vi "RabiMeasurement.vi"() -> ()   [LabVIEW 2020]
uses:
  <vilib>/Swabian Instruments/Pulse Streamer/PulseStreamer/PulseStreamer/typedefs/typedef_TriggerStart.ctl
  <vilib>/Swabian Instruments/Pulse Streamer/PulseStreamer/PulsePattern/PulsePattern.lvclass
  C:/Program Files (x86)/National Instruments/LabVIEW 2020/vi.lib/Swabian Instruments/Pulse Streamer/PulseStreamer/Pattern/Pattern.lvclass
  <vilib>/Swabian Instruments/Pulse Streamer/PulseStreamer/typedefs/typedef_ChannelNumber.ctl
  <vilib>/Swabian Instruments/Pulse Streamer/PulseStreamer/AnalogPattern/AnalogPattern.lvclass
  <vilib>/Swabian Instruments/Pulse Streamer/PulseStreamer/Sequence/Sequence.lvclass/Sequence.ctl
  <vilib>/Analysis/baseanly.llb/Mean (DBL).vi
  <vilib>/FPGAPlugInAG/USB-7855R/niLvFpga_Open_USB-7855R.vi
  <vilib>/rvi/interface/common/dynamic/niFpgaDynamicAddResources.vi
  <vilib>/rvi/interface/common/niFpgaWaitOnOcc.vi
  <vilib>/Utility/error.llb/Error Cluster From Error Code.vi
  <vilib>/Swabian Instruments/Pulse Streamer/PulseStreamer/Pattern/Read total duration.vi
  <vilib>/Swabian Instruments/Pulse Streamer/PulseStreamer/PulseStreamer/stream/stream (Sequence).vi
  <vilib>/rvi/errors/niLvFpgaAdjustHostInterfaceError.vi
  <vilib>/FPGAPlugInAG/Dynamic/niLvFpga_Close_Dynamic.vi
  <vilib>/rvi/interface/nirviOpenFPGA/nirviOpenFPGA.xnode
  FPGA Bitfiles/pulsedcodespract_FPGATarget_FPGAReadout_kZLwuzG+bY8.lvbitx
  <vilib>/rvi/interface/nirviMethod/nirviMethod.xnode
  <vilib>/rvi/interface/nirviCloseFPGA/nirviCloseFPGA.xnode
  <vilib>/Swabian Instruments/Pulse Streamer/PulseStreamer/PulseStreamer/PulseStreamer.lvclass
  <vilib>/Swabian Instruments/Pulse Streamer/PulseStreamer/Sequence/Sequence.lvclass
  <vilib>/FPGAPlugInAG/Dynamic/niLvFpga_ConfigureFifo_Dynamic.vi
  <vilib>/rvi/errors/niLvFpgaMergeErrorWithErrorCode.vi
  <vilib>/Swabian Instruments/Pulse Streamer/PulseStreamer/PulseStreamer.lvlib
  <vilib>/FPGAPlugInAG/Dynamic/niLvFpga_ReadFifo_Dynamic.vi
  <vilib>/Analysis/NI_AALBase.lvlib
panel:
  in  "532 AOM Voltage":dbl min=-1.0 max=1.0
  in  "Pulser Start":T1
  out "Elements Remaining":dbl
  out "Cycle Num":i32
  in  "Delay(ns)":i32=760
  out "Seq Duration(ms)":dbl
  out "size(s)":dbl
  out "n_runs":i32
  out "Tau Set":i32
  out "Exp Number":i32
  in  "IP PulseBlaster":string="169.254.8.2"
  in  "Cycles":i32
  in  "Tau Step(ns)":i32=1
  in  "Tau Start(ns)":i32=5
  in  "Expt Repeat":u32=1000
  in  "Repeat":i32=10
  in  "Pulse Num":i32=100000
  in  "Wait Time(ns)":i32=600
  in  "Readout (ns)":i32=200
  in  "Initialization time (ns)":i32=1000
  out "ESR Plot Avg":cluster{"Tau":i32[], dbl[]}(graph)
  out "AvgCountsTrack":cluster{"Tau":i32[], dbl[]}(graph)
  out "Averaged_ESR":dbl[](array[numeric])
  out "AverageCounts This Run":cluster{"N_array":i32[], "CountAverage":dbl[]}(graph)
  out "Count_Track":dbl[](array[numeric])
  out "N_array":i32[](array[numeric])
  out "CountAverage":dbl[](array[numeric])
  out "ESR Plot Current Run":cluster{"Tau":i32[], "ESR Data":dbl[]}(graph)
  out "Counts":cluster{"Tau":i32[], "Count":u32[]}(graph)
  out "Tau":i32[](array[numeric])
  out "ESR Data":dbl[](array[numeric])
  out "Count":u32[](array[numeric])
  out "Digital plot":cluster{"CumTime":i64[], dbl[]}[](graph)
  out "RF Freq Set(GHz)":dbl format="%_8g"
  in  "RF Power (dBm)":dbl=1000000000.0 format="%_4g"
  in  "RF Freq(Hz)":dbl=1000000000.0 format="%_8g"
  in  "GPIB Reference":string="1:27"
  in  "?":bool
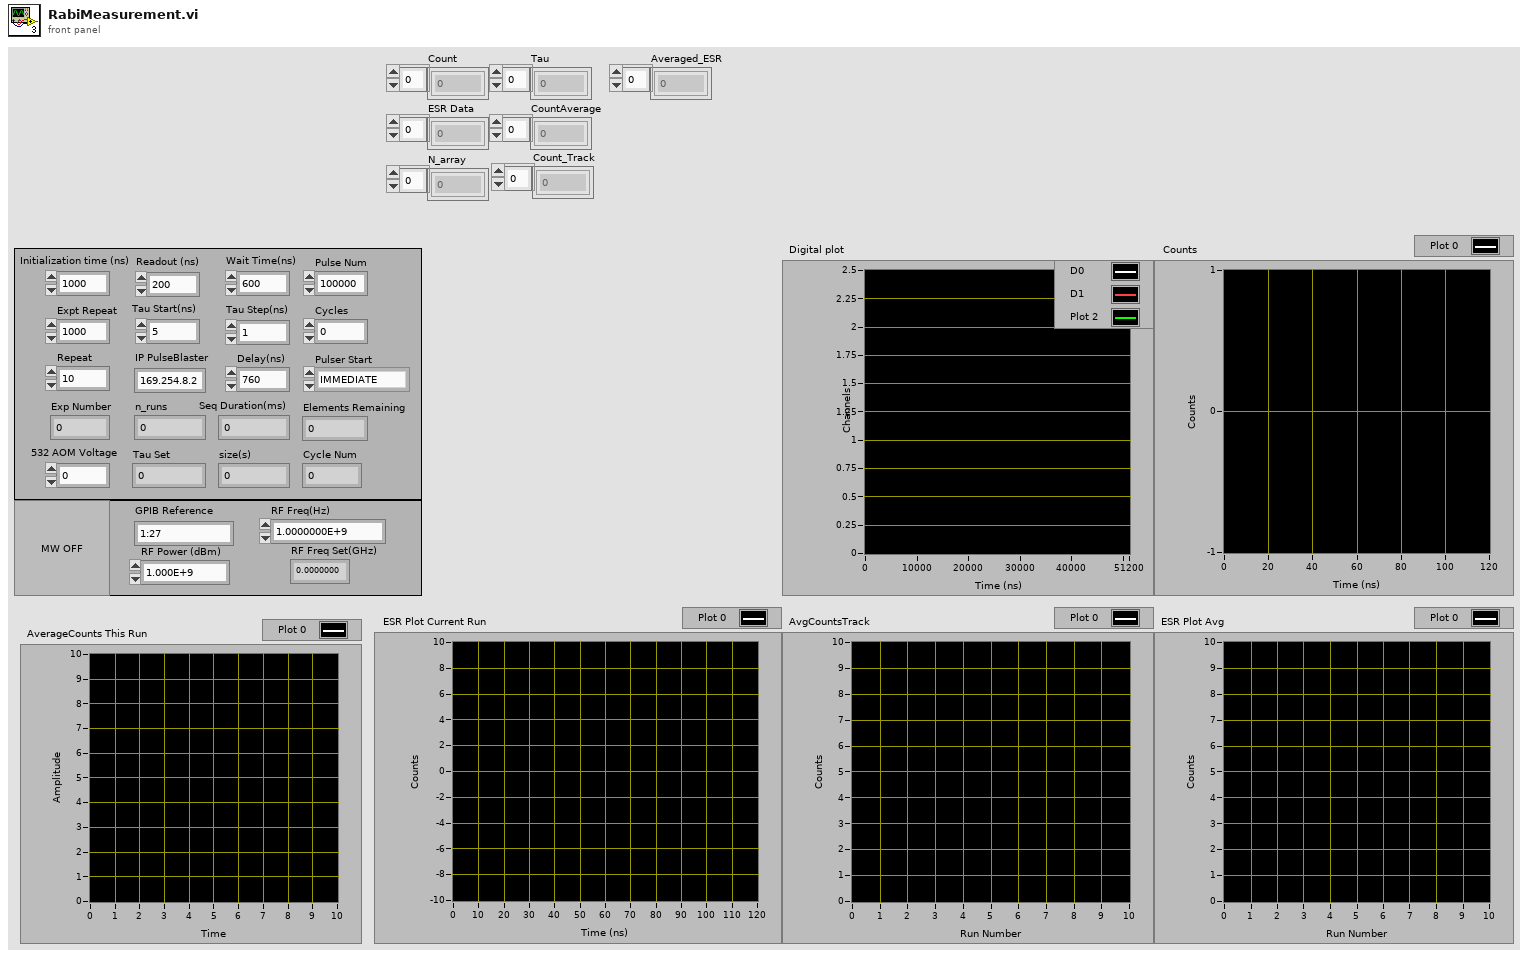
[diagram p1: front panel]
types:
  T1 = typedef "PulseStreamer.lvlib/PulseStreamer.lvclass/typedef_TriggerStart.ctl" = enum16{"IMMEDIATE", "SOFTWARE", "HW_RISING", "HW_FALLING", "HW_RISING_AND_FALLING"}
  T2 = typedef "PulseStreamer.lvlib/typedef_ChannelNumber.ctl" = i16
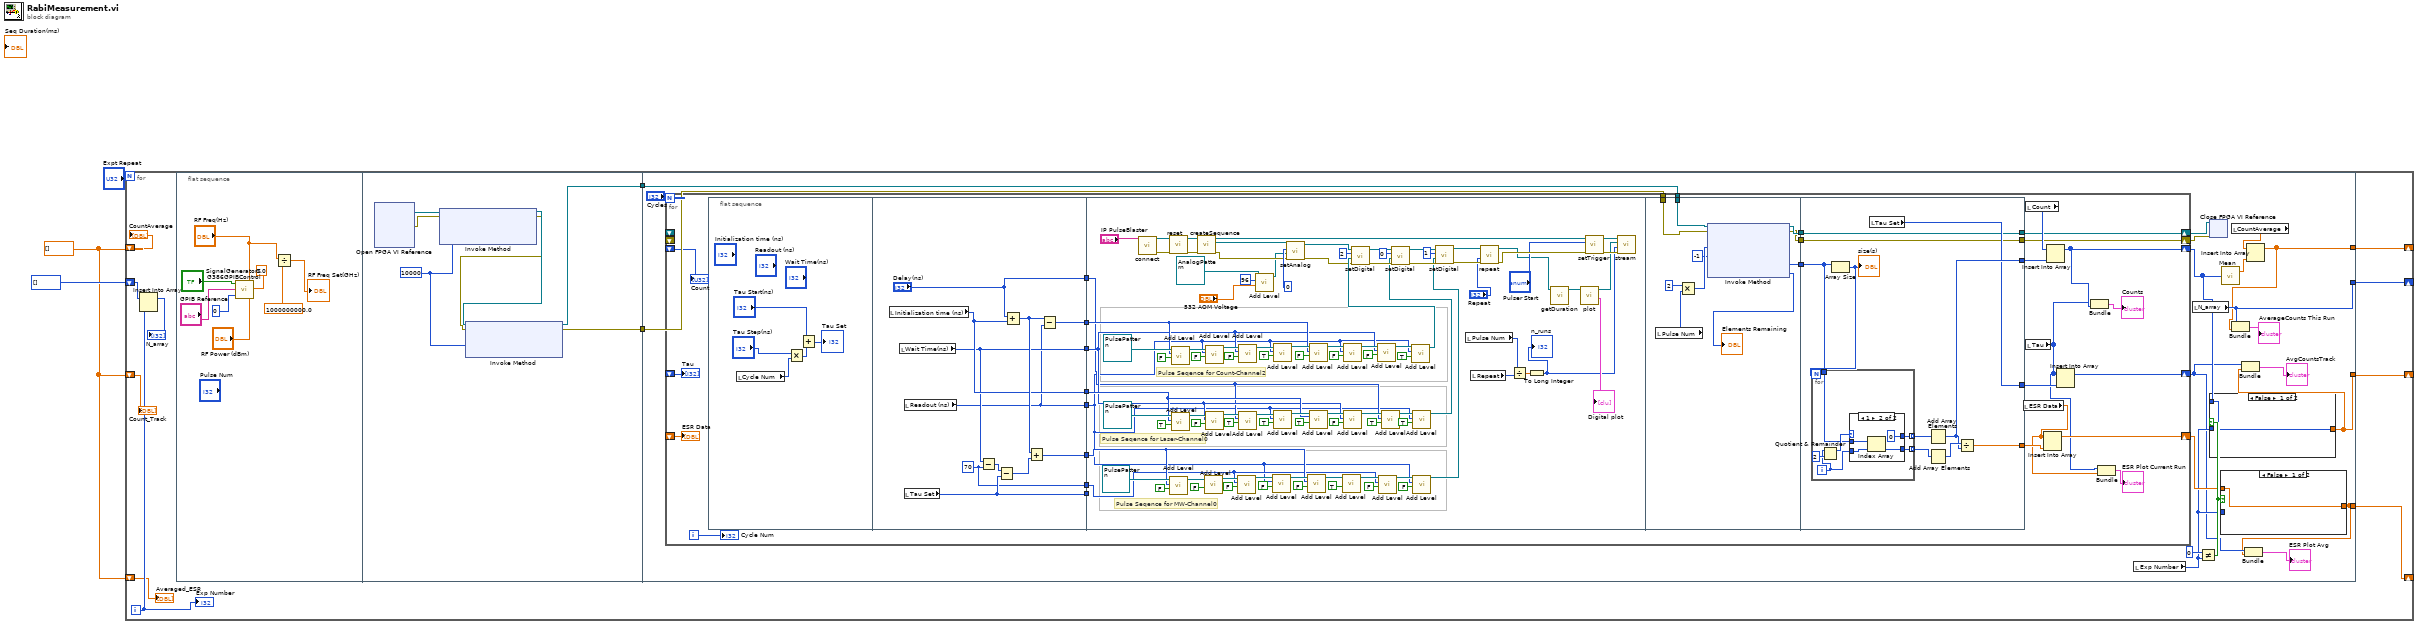
[diagram p0: block diagram]
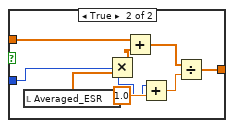
[diagram p2: hidden frame]
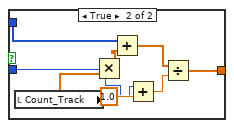
[diagram p3: hidden frame]
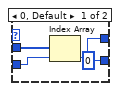
[diagram p4: hidden frame]
diagram:
  w1 = dbl[] []
  n1 = for {
    N: "Expt Repeat" -> [_]
    shift-right: [w13] -> _
    shift-left: w1 -> [w12]
    shift-right: [w8] -> _
    shift-left: i32[] [] -> [w11]
    shift-right: [w6] -> _
    shift-left: w1 -> [w9]
    shift-right: [w4] -> _
    shift-left: w1 -> [w5]
    i -> [w7]
    n2 = Insert Into Array(array=w11, new element=w7) -> (→"N_array":i32[])  [unwired: 1 in]
    n3 = flat-sequence {
      tunnel: [w25] -> w15
      tunnel: [w24] -> w14
      tunnel: w15 -> [w49]
      tunnel: w14 -> [w48]
      tunnel: [w42] -> w13
      tunnel: [w43] -> w8
      tunnel: [w36] -> w6
      tunnel: [w32] -> w4
      frame #0 {
        n4 = call "SignalGeneratorSG386GPIBControl.vi"("RF Power (dBm)"="RF Power (dBm)", "RF Freq Step (Hz)"=0.0, "RF Freq (Hz)"="RF Freq(Hz)", "Current loop"=0, "GPIB RF"="GPIB Reference", "uWave Enable"="?") -> ()
        n5 = Divide(x="RF Freq(Hz)", y=1000000000.0) -> (x/y=→"RF Freq Set(GHz)":dbl)
      }
      frame #1 {
        w26 = u32 10000 ("Requested Depth")
        n6 = xnode "Open FPGA VI Reference"() -> ("FPGA VI Reference Out"=w30:refnum<k20>, "error out"=w29:errorcluster)  [unwired: 2 in]
        n7 = xnode "Invoke Method"("FPGA VI Reference In"=w30, "error in"=w29, "Requested Depth"=w26) -> ("FPGA VI Reference Out"=w28:refnum<k20>, "error out"=w27:errorcluster)  [unwired: 1 out]
        n8 = xnode "Invoke Method"("FPGA VI Reference In"=w28, "error in"=w27, "Requested Depth"=w26) -> ("FPGA VI Reference Out"=w25:refnum<k20>, "error out"=w24:errorcluster)  [unwired: 1 out]
      }
      frame #2 {
        n9 = for {
          N: "Cycles" -> [_]
          tunnel: w49 -> [w89]
          tunnel: w48 -> [w88]
          shift-right: [w77] -> w39
          shift-left: _ -> [w84]
          shift-right: [w82] -> w38
          shift-left: _ -> [w81]
          shift-right: [w79] -> w33
          shift-left: _ -> [w78]
          shift-right: [w71] -> w47
          shift-left: _ -> [_]
          shift-right: [w69] -> w46
          shift-left: _ -> [_]
          i -> [w98]
          n10 = flat-sequence {
            tunnel: [w114] -> w97
            tunnel: [w110] -> w96
            tunnel: ["Delay(ns)"] -> w95
            tunnel: [w108] -> w94
            tunnel: [w107] -> w93
            tunnel: [w106] -> w92
            tunnel: [w105] -> w91
            tunnel: [w104] -> w90
            tunnel: w97 -> [w164]
            tunnel: w96 -> [w152]
            tunnel: w95 -> [w157]
            tunnel: w94 -> [w159]
            tunnel: w93 -> [w158]
            tunnel: w92 -> [w150]
            tunnel: w91 -> [_]
            tunnel: w90 -> [w151]
            tunnel: w89 -> [w219]
            tunnel: w88 -> [w218]
            tunnel: [w212] -> w87
            tunnel: [w211] -> w72
            tunnel: [w210] -> w70
            tunnel: w87 -> [w228]
            tunnel: [w224] -> w86
            tunnel: [w223] -> w83
            tunnel: [w222] -> w80
            tunnel: [w221] -> w71
            tunnel: w72 -> [w221]
            tunnel: w70 -> [w220]
            tunnel: [w220] -> w69
            frame #0 {
              n11 = local read "Cycle Num"() -> (w103:i32)
              n12 = Multiply(x="Tau Step(ns)", y=w103) -> (x*y=w101:i32)
              n13 = Add(x="Tau Start(ns)", y=w101) -> (x+y=→"Tau Set":i32)
            }
            frame #1 {
              w104 = 70 ("y")
              n14 = local read "Initialization time (ns)"() -> (w108:i32)
              n15 = local read "Wait Time(ns)"() -> (w107:i32)
              n16 = local read "Readout (ns)"() -> (w106:i32)
              n17 = local read "Tau Set"() -> (w105:i32)
              n18 = Subtract(x=w107, y=w104) -> (x-y=w111:i32)
              n19 = Subtract(x=w111, y=w105) -> (x-y=w112:i32)
              n20 = Add(x="Delay(ns)", y=w108) -> (x+y=w113:i32)
              n21 = Add(x=w113, y=w112) -> (x+y=w110:i32)
              n22 = Subtract(x=w113, y=w106) -> (x-y=w114:i32)
            }
            frame #2 {
              # "Pulse Seqence for MW-Channel0"
              # "Pulse Seqence for Laser-Channel0"
              # "Pulse Seqence for Count-Channel2"
              n23 = call <vilib>:"connect.vi"("ip"="IP PulseBlaster") -> ("error out"=w208:errorcluster, "Pulse Streamer out"=w207:refnum<class "PulseStreamer.lvclass">)  [unwired: 9 in]
              n24 = call <vilib>:"reset.vi"("error in (no error)"=w208, "Pulse Streamer in"=w207) -> ("error out"=w206:errorcluster, "Pulse Streamer out"=w205:refnum<class "PulseStreamer.lvclass">)  [unwired: 8 in]
              n25 = call <vilib>:"Add Level.vi"("Level"=FALSE, "Duration"=w152, "Digital Sequence in"=refnum<class "PulsePattern.lvclass"> refnum) -> ("Digital Sequence out"=w173:refnum<class "PulsePattern.lvclass">)  [unwired: 8 in]
              n26 = call <vilib>:"Add Level.vi"("Level"=FALSE, "Duration"=w164, "Digital Sequence in"=refnum<class "PulsePattern.lvclass"> refnum) -> ("Digital Sequence out"=w201:refnum<class "PulsePattern.lvclass">)  [unwired: 8 in]
              n27 = call <vilib>:"Add Level.vi"("Level"=TRUE, "Duration"=w159, "Digital Sequence in"=refnum<class "PulsePattern.lvclass"> refnum) -> ("Digital Sequence out"=w180:refnum<class "PulsePattern.lvclass">)  [unwired: 8 in]
              n28 = call-dynamic "createSequence.vi"("error in (no error)"=w206, "PulseStreamer in"=w205) -> ("error out"=w122:errorcluster, "Sequence"=w116:refnum<class "Sequence.lvclass">, "PulseStreamer out"=w136:refnum<class "PulseStreamer.lvclass">)  [unwired: 7 in]
              n29 = call <vilib>:"Add Level.vi"("Level"=FALSE, "Digital Sequence in"=w173) -> ("Digital Sequence out"=w171:refnum<class "PulsePattern.lvclass">)  [unwired: 9 in]
              n30 = call <vilib>:"Add Level.vi"("Level"=FALSE, "Duration"=w150, "Digital Sequence in"=w201) -> ("Digital Sequence out"=w199:refnum<class "PulsePattern.lvclass">)  [unwired: 8 in]
              n31 = call <vilib>:"Add Level.vi"("Level"=FALSE, "Duration"=w158, "Digital Sequence in"=w180) -> ("Digital Sequence out"=w182:refnum<class "PulsePattern.lvclass">)  [unwired: 8 in]
              n32 = call <vilib>:"Add Level.vi"("Level"=FALSE, "Duration"=w151, "Digital Sequence in"=w171) -> ("Digital Sequence out"=w169:refnum<class "PulsePattern.lvclass">)  [unwired: 8 in]
              n33 = call <vilib>:"Add Level.vi"("Level"=FALSE, "Duration"=w158, "Digital Sequence in"=w199) -> ("Digital Sequence out"=w197:refnum<class "PulsePattern.lvclass">)  [unwired: 8 in]
              n34 = call <vilib>:"Add Level.vi"("Level"=TRUE, "Duration"=w157, "Digital Sequence in"=w182) -> ("Digital Sequence out"=w184:refnum<class "PulsePattern.lvclass">)  [unwired: 8 in]
              n35 = call <vilib>:"Add Level.vi"("Voltage"="532 AOM Voltage", "Duration"=i64 96, "Analog Sequence in"=refnum<class "AnalogPattern.lvclass"> refnum) -> ("Analog Sequence out"=w117:refnum<class "AnalogPattern.lvclass">)  [unwired: 8 in]
              n36 = call <vilib>:"Add Level.vi"("Level"=FALSE, "Duration"=w150, "Digital Sequence in"=w169) -> ("Digital Sequence out"=w167:refnum<class "PulsePattern.lvclass">)  [unwired: 8 in]
              n37 = call <vilib>:"Add Level.vi"("Level"=TRUE, "Duration"=w150, "Digital Sequence in"=w197) -> ("Digital Sequence out"=w195:refnum<class "PulsePattern.lvclass">)  [unwired: 8 in]
              n38 = call <vilib>:"Add Level.vi"("Level"=TRUE, "Duration"=w150, "Digital Sequence in"=w184) -> ("Digital Sequence out"=w186:refnum<class "PulsePattern.lvclass">)  [unwired: 8 in]
              n39 = call-dynamic "setAnalog.vi"("error in (no error)"=w122, "AnalogPattern"=w117, "channel"=T2 0, "Sequence in"=w116) -> ("error out"=w121:errorcluster, "Sequence out"=w115:refnum<class "Sequence.lvclass">)  [unwired: 6 in]
              n40 = call <vilib>:"Add Level.vi"("Level"=FALSE, "Duration"=w152, "Digital Sequence in"=w167) -> ("Digital Sequence out"=w165:refnum<class "PulsePattern.lvclass">)  [unwired: 8 in]
              n41 = call <vilib>:"Add Level.vi"("Level"=FALSE, "Duration"=w164, "Digital Sequence in"=w195) -> ("Digital Sequence out"=w193:refnum<class "PulsePattern.lvclass">)  [unwired: 8 in]
              n42 = call <vilib>:"Add Level.vi"("Level"=TRUE, "Duration"=w159, "Digital Sequence in"=w186) -> ("Digital Sequence out"=w188:refnum<class "PulsePattern.lvclass">)  [unwired: 8 in]
              n43 = call <vilib>:"Add Level.vi"("Level"=TRUE, "Digital Sequence in"=w165) -> ("Digital Sequence out"=w153:refnum<class "PulsePattern.lvclass">)  [unwired: 9 in]
              n44 = call <vilib>:"Add Level.vi"("Level"=FALSE, "Duration"=w150, "Digital Sequence in"=w193) -> ("Digital Sequence out"=w191:refnum<class "PulsePattern.lvclass">)  [unwired: 8 in]
              n45 = call <vilib>:"Add Level.vi"("Level"=FALSE, "Duration"=w158, "Digital Sequence in"=w188) -> ("Digital Sequence out"=w160:refnum<class "PulsePattern.lvclass">)  [unwired: 8 in]
              n46 = call <vilib>:"Add Level.vi"("Level"=FALSE, "Duration"=w158, "Digital Sequence in"=w191) -> ("Digital Sequence out"=w189:refnum<class "PulsePattern.lvclass">)  [unwired: 8 in]
              n47 = call <vilib>:"Add Level.vi"("Level"=FALSE, "Duration"=w151, "Digital Sequence in"=w153) -> ("Digital Sequence out"=w156:refnum<class "PulsePattern.lvclass">)  [unwired: 8 in]
              n48 = call <vilib>:"Add Level.vi"("Level"=TRUE, "Duration"=w157, "Digital Sequence in"=w160) -> ("Digital Sequence out"=w161:refnum<class "PulsePattern.lvclass">)  [unwired: 8 in]
              n49 = call <vilib>:"Add Level.vi"("Level"=TRUE, "Duration"=w150, "Digital Sequence in"=w189) -> ("Digital Sequence out"=w148:refnum<class "PulsePattern.lvclass">)  [unwired: 8 in]
              n50 = call-dynamic "setDigital.vi"("error in (no error)"=w121, "PulsePattern"=w148, "channel"=T2 2, "Sequence in"=w115) -> ("error out"=w143:errorcluster, "Sequence out"=w147:refnum<class "Sequence.lvclass">)  [unwired: 6 in]
              n51 = call <vilib>:"Add Level.vi"("Level"=TRUE, "Duration"=w150, "Digital Sequence in"=w161) -> ("Digital Sequence out"=w141:refnum<class "PulsePattern.lvclass">)  [unwired: 8 in]
              n52 = call-dynamic "setDigital.vi"("error in (no error)"=w143, "PulsePattern"=w141, "channel"=T2 0, "Sequence in"=w147) -> ("error out"=w142:errorcluster, "Sequence out"=w146:refnum<class "Sequence.lvclass">)  [unwired: 6 in]
              n53 = call <vilib>:"Add Level.vi"("Level"=FALSE, "Duration"=w150, "Digital Sequence in"=w156) -> ("Digital Sequence out"=w140:refnum<class "PulsePattern.lvclass">)  [unwired: 8 in]
              n54 = call-dynamic "setDigital.vi"("error in (no error)"=w142, "PulsePattern"=w140, "channel"=T2 1, "Sequence in"=w146) -> ("error out"=w139:errorcluster, "Sequence out"=w138:refnum<class "Sequence.lvclass">)  [unwired: 6 in]
              n55 = local read "Pulse Num"() -> (w127:i32)
              n56 = local read "Repeat"() -> (w126:i32)
              n57 = call <vilib>:"repeat.vi"("error in (no error)"=w139, "Repeat count"="Repeat", "Sequence in"=w138) -> ("error out"=w135:errorcluster, "Sequence out"=w130:refnum<class "Sequence.lvclass">)  [unwired: 7 in]
              n58 = Divide(x=w127, y=w126) -> (x/y=w125:dbl)
              n59 = To Long Integer(number=w125) -> (32bit integer=w124:i32)
              "n_runs" <- w124
              n60 = call <vilib>:"getDuration.vi"("Sequence in"=w130) -> ("Sequence out"=w131:refnum<class "Sequence.lvclass">)  [unwired: 9 in, 1 out]
              n61 = call <vilib>:"plot.vi"("Sequence in"=w131) -> ("Digital plot"=→"Digital plot":cluster{"CumTime":i64[], dbl[]}[], "Sequence out"=w129:refnum<class "Sequence.lvclass">)  [unwired: 7 in, 2 out]
              n62 = call-dynamic "setTrigger.vi"("error in (no error)"=w135, "start"="Pulser Start", "Pulse Streamer in"=w136) -> ("error out"=w133:errorcluster, "Pulse Streamer out"=w132:refnum<class "PulseStreamer.lvclass">)  [unwired: 7 in]
              n63 = call-poly <vilib>:"stream.vi"("error in (no error)"=w133, "n_runs"=w124, "sequence"=w129, "Pulse Streamer in"=w132) -> ()  [unwired: 4 in, 2 out]
            }
            frame #3 {
              n64 = local read "Pulse Num"() -> (w217:i32)
              n65 = Multiply(x=2, y=w217) -> (x*y=w215:i32)
              n66 = xnode "Invoke Method"("FPGA VI Reference In"=w219, "error in"=w218, "Number of Elements"=w215, "Timeout (ms)"=-1) -> ("FPGA VI Reference Out"=w211:refnum<k20>, "error out"=w210:errorcluster, "Data"=w212:u32[], "Elements Remaining"=→"Elements Remaining":u32)
            }
            frame #4 {
              n67 = Array Size(array=w228) -> (size(s)=w229:i32)
              "size(s)" <- w229
              n68 = for {
                N: w229 -> [_]
                tunnel: w228 -> [w232]
                tunnel: [w231] -> w227 mode=indexing
                tunnel: [w230] -> w226 mode=indexing
                i -> [w233]
                n69 = Quotient & Remainder(x=w233, y=2) -> (x-y*floor(x/y)=w234:i32)  [unwired: 1 out]
                n70 = case shown="1" w234 {
                  tunnel: w233 -> [w239 w243]
                  tunnel: w232 -> [w238 w242]
                  tunnel: [u32 0 w241] -> w231
                  tunnel: [w237 u32 0] -> w230
                  frame 0, Default {
                    n71 = Index Array(array=w238, index=w239) -> (element=w237:u32)
                  }
                  frame 1 {
                    n72 = Index Array(array=w242, index=w243) -> (element=w241:u32)
                  }
                }
              }
              n73 = local read "Tau Set"() -> (w222:i32)
              n74 = Add Array Elements(numeric array=w226) -> (sum=w224:u32)
              n75 = Add Array Elements(numeric array=w227) -> (sum=w225:u32)
              n76 = Divide(x=w225, y=w224) -> (x/y=w223:dbl)
            }
          }
          n77 = local read "ESR Data"() -> (w74:dbl[])
          n78 = local read "Count"() -> (w85:u32[])
          n79 = local read "Tau"() -> (w75:i32[])
          n80 = Insert Into Array(array=w74, new element=w83) -> (w82:dbl[])  [unwired: 1 in]
          n81 = Insert Into Array(array=w85, new element=w86) -> (w77:u32[])  [unwired: 1 in]
          n82 = Insert Into Array(array=w75, new element=w80) -> (w79:i32[])  [unwired: 1 in]
          n83 = Bundle("Tau"=w75, "Count"=w77) -> (→"Counts":cluster{"Tau":i32[], "Count":u32[]})  [unwired: 1 in]
          n84 = Bundle("Tau"=w75, "ESR Data"=w74) -> (→"ESR Plot Current Run":cluster{"Tau":i32[], "ESR Data":dbl[]})  [unwired: 1 in]
          "Cycle Num" <- w98
          "Count" <- w84
          "ESR Data" <- w81
          "Tau" <- w78
        }
        n85 = local read "Exp Number"() -> (w37:i32)
        n86 = local read "N_array"() -> (w43:i32[])
        n87 = Not Equal?(x=0, y=w37) -> (x != y?=w40:bool)
        n88 = xnode "Close FPGA VI Reference"("FPGA VI Reference In"=w47, "error in"=w46) -> ()  [unwired: 1 out]
        n89 = case shown="False" w40 {
          tunnel: w37 -> [_ w63]
          tunnel: w39 -> [w60 w67]
          tunnel: [w60 w62] -> w36
          frame False {
          }
          frame True {
            n90 = local read "Count_Track"() -> (w68:dbl[])
            n91 = Multiply(x=w63, y=w68) -> (x*y=w66:dbl[])
            n92 = Add(x=w67, y=w66) -> (x+y=w61:dbl[])
            n93 = Add(x=w63, y=1.0) -> (x+y=w65:dbl)
            n94 = Divide(x=w61, y=w65) -> (x/y=w62:dbl[])
          }
        }
        n95 = case shown="False" w40 {
          tunnel: w38 -> [w51 w54]
          tunnel: w37 -> [_ w53]
          tunnel: [w51 w52] -> w32
          frame False {
          }
          frame True {
            n96 = local read "Averaged_ESR"() -> (w55:dbl[])
            n97 = Multiply(x=w53, y=w55) -> (x*y=w56:dbl[])
            n98 = Add(x=w54, y=w56) -> (x+y=w59:dbl[])
            n99 = Add(x=w53, y=1.0) -> (x+y=w57:dbl)
            n100 = Divide(x=w59, y=w57) -> (x/y=w52:dbl[])
          }
        }
        n101 = call-poly <vilib>:"Mean.vi"("X"=w39) -> ("mean"=w31:dbl)  [unwired: 1 out]
        n102 = local read "CountAverage"() -> (w45:dbl[])
        n103 = Bundle("Tau"=w33, "Count"=w36) -> (→"AvgCountsTrack":cluster{"Tau":i32[], "Count":dbl[]})  [unwired: 1 in]
        n104 = Bundle("Tau"=w33, "ESR Data"=w32) -> (→"ESR Plot Avg":cluster{"Tau":i32[], "ESR Data":dbl[]})  [unwired: 1 in]
        n105 = Insert Into Array(array=w45, new element=w31) -> (w42:dbl[])  [unwired: 1 in]
        n106 = Bundle("N_array"=w43, "CountAverage"=w42) -> (→"AverageCounts This Run":cluster{"N_array":i32[], "CountAverage":dbl[]})  [unwired: 1 in]
      }
    }
    "CountAverage" <- w12
    "Count_Track" <- w9
    "Exp Number" <- w7
    "Averaged_ESR" <- w5
  }
